vi "OP600ZP_INTLCK_LOOP.vi"(8 "errin":errorcluster caption="entrée d'erreur (pas d'erreur)") -> (0 "errout":errorcluster caption="sortie d'erreur", 2 "pass?":bool, 3 "Logout":string)   [LabVIEW 2020]
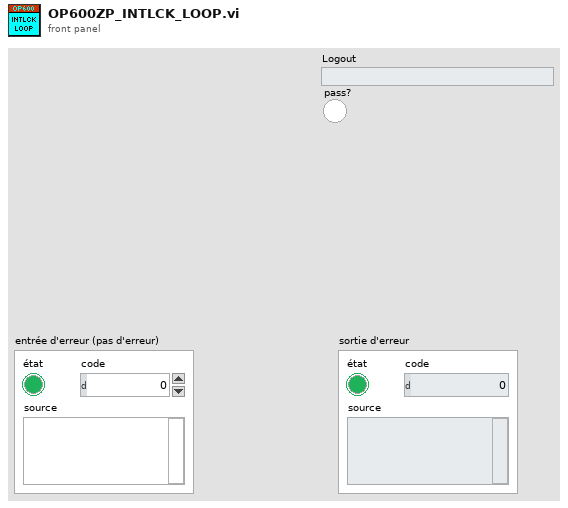
[diagram p1: front panel]
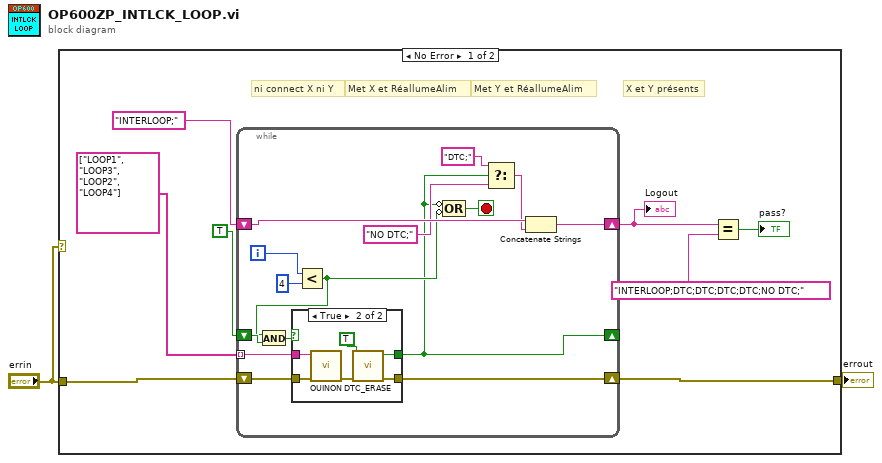
[diagram p0: block diagram]
diagram:
  n1 = case shown="No Error" "errin" {
    tunnel: "errin" -> [w9 w33]
    tunnel: [w6 w33] -> w2
    frame No Error {
      # "X et Y présents"
      # "Met Y et RéallumeAlim"
      # "Met X et RéallumeAlim"
      # "ni connect X ni Y"
      n2 = while {
        tunnel: string[] ["LOOP1", "LOOP3", "LOOP2", "LOOP4"] -> [w25] mode=indexing
        shift-right: [w23] -> w6
        shift-left: w9 -> [w24]
        shift-right: [w11] -> _
        shift-left: TRUE -> [w14]
        shift-right: [w19] -> w5
        shift-left: "INTERLOOP;" ("chaîne") -> [w20]
        i -> [w12]
        stop <- w22 stop-if-true
        n3 = Less?(x=w12, y=4) -> (x < y?=w13:bool)
        n4 = And(x=w13, y=w14) -> (x .and. y?=w15:bool)
        n5 = case shown="True" w15 {
          tunnel: w25 -> [_ w32]
          tunnel: w24 -> [w26 w30]
          tunnel: [w26 w29] -> w23
          tunnel: [_ w28] -> w11
          frame False {
          }
          frame True {
            n6 = call "OUINON.vi"("errin"=w30, "image"=w32) -> ("error out"=w31:errorcluster)  [unwired: 8 in, 1 out]
            n7 = call "DTC_ERASE.vi"("errin"=w31, "UNINIT?"=TRUE) -> ("error out"=w29:errorcluster, "Erased?"=w28:bool)  [unwired: 8 in]
          }
        }
        n8 = Compound Arithmetic op=OR(invert w11, invert w13) -> (w22:bool)
        n9 = Select(t="DTC;", s=w11, f="NO DTC;") -> (s? t:f=w16:string)
        n10 = Concatenate Strings(w20, w16) -> (w19:string)
      }
      "Logout" <- w5
      n11 = Equal?(x=w5, y="INTERLOOP;DTC;DTC;DTC;DTC;NO DTC;") -> (x = y?=→"pass?":bool)
    }
    frame Error {
    }
  }
  "errout" <- w2
